vi "GFITS_GetQueued.vi"(10 "input":string) -> (1 "queued?":bool, 2 "output":string)   [LabVIEW 2016]
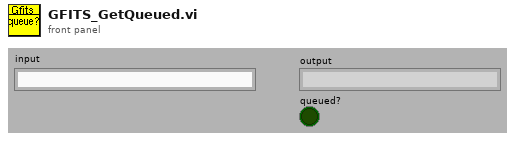
[diagram p1: front panel]
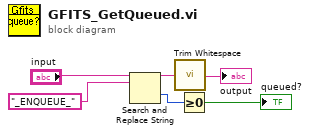
[diagram p0: block diagram]
diagram:
  n1 = Search and Replace String(input string="input", search string="_ENQUEUE_") -> (result string=w4:string, offset past replacement=w3:i32)  [unwired: 1 in, 7 out]
  n2 = call <vilib>:"Trim Whitespace.vi"("string"=w4) -> ("trimmed string"=→"output":string)  [unwired: 1 in]
  n3 = Greater Or Equal To 0?(x=w3) -> (x >= 0?=→"queued?":bool)
